vi "Workshop Exercise 2 Solution.vi"() -> ()   [LabVIEW 2019]
panel:
  in  "Enqueue Speed [ms]":u32=100
  in  "Dequeue Speed [ms]":u32=100
  out "Received Elements":dbl(graph)
  out "Generated Elements":dbl(graph)
  out "Elements in Queue":i32(slide) scale=0.0..100.0
  in  "Stop":bool
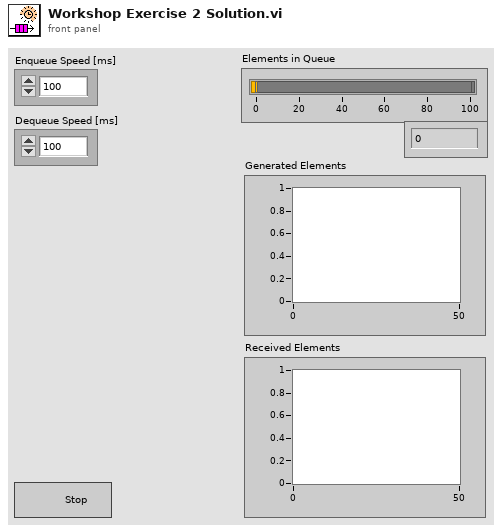
[diagram p1: front panel]
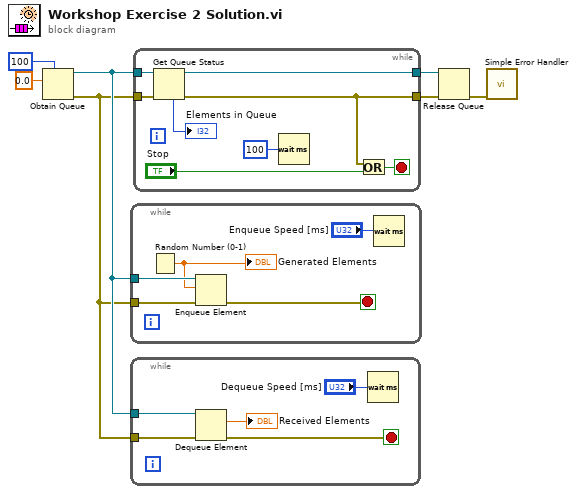
[diagram p0: block diagram]
diagram:
  n1 = Obtain Queue(max queue size (-1, unlimited)=100 ("max queue size"), element data type=0.0) -> (queue out=w7:refnum<queue>, error out=w6:errorcluster)  [unwired: 3 in, 1 out]
  n2 = while {
    tunnel: w7 -> [w12]
    tunnel: w6 -> [w11]
    stop <- w10 stop-if-true
    # "Enqueue Loop"
    n3 = Random Number (0-1)() -> (number: 0 to 1=w9:dbl)
    "Generated Elements" <- w9
    n4 = Enqueue Element(queue=w12, element=w9, error in (no error)=w11) -> (error out=w10:errorcluster)  [unwired: 3 out]
    n5 = Wait (ms)(milliseconds to wait="Enqueue Speed [ms]") -> ()  [unwired: 1 out]
  }
  n6 = while {
    tunnel: w7 -> [w17]
    tunnel: w6 -> [w16]
    stop <- w15 stop-if-true
    # "Dequeue Loop"
    n7 = Dequeue Element(queue=w17, error in (no error)=w16) -> (element=→"Received Elements":dbl, error out=w15:errorcluster)  [unwired: 3 out]
    n8 = Wait (ms)(milliseconds to wait="Dequeue Speed [ms]") -> ()  [unwired: 1 out]
  }
  n9 = while {
    tunnel: w7 -> [w25]
    tunnel: [w19] -> w5
    tunnel: w6 -> [w21]
    tunnel: [w20] -> w4
    stop <- w23 stop-if-true
    # "Queue Status"
    n10 = Get Queue Status(queue=w25, error in (no error)=w21) -> (queue out=w20:refnum<queue>, error out=w19:errorcluster, # elements in queue=→"Elements in Queue":i32)  [unwired: 6 out]
    n11 = Wait (ms)(milliseconds to wait=u32 100) -> ()  [unwired: 1 out]
    n12 = Or(x=w19, y="Stop") -> (x .or. y?=w23:bool)
  }
  n13 = Release Queue(queue=w4, error in (no error)=w5) -> (error out=w3:errorcluster)  [unwired: 3 out]
  n14 = call <vilib>:"Simple Error Handler.vi"("error in (no error)"=w3) -> ()  [unwired: 1 in, 8 out]
